vi "Elevator Settled.vi"(8 "error in (no error)":errorcluster, 10 "State":T1=enum."Tote 1", 11 "Elevator Inputs":T2={"Up"=FALSE, "Down"=FALSE, "Bin Modifier"=FALSE, "Pickup"=FALSE, "Top LS"=FALSE, "Bottom LS"=FALSE, "Encoder Position"=-460.0, "Encoder Velocity"=0.0, "Manual Control"=0.0}) -> (0 "error out":errorcluster, 2 "Settled?":bool, 3 "State":T1=enum."Tote 1")   [LabVIEW 2014]
uses:
  Elevator Input Data.ctl
  Elevator States.ctl
panel:
  in  "Velocity\nTolerance":dbl=300000000.0
  in  "Position\nTolerance":dbl=50.0
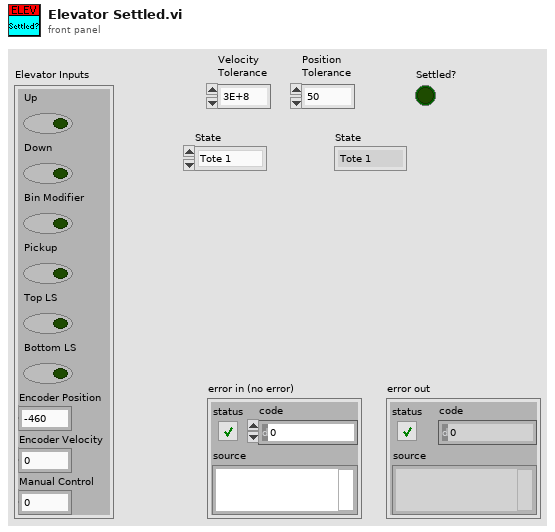
[diagram p1: front panel]
types:
  T1 = typedef "Elevator States.ctl" = enum16{"Ground", "Tote 1", "Tote 2", "Tote 3", "Tote 4", "Tote 5", "Tote 6"}
  T2 = typedef "Elevator Input Data.ctl" = cluster{"Up":bool, "Down":bool, "Bin Modifier":bool, "Pickup":bool, "Top LS":bool, "Bottom LS":bool, "Encoder Position":dbl, "Encoder Velocity":dbl, "Manual Control":dbl}
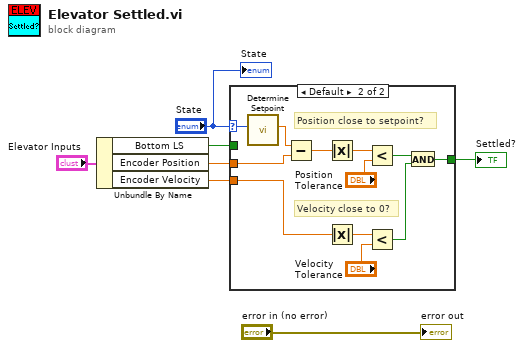
[diagram p0: block diagram]
diagram:
  n1 = Unbundle By Name("Elevator Inputs") -> ("Bottom LS"=w6:bool, "Encoder Position"=w5:dbl, "Encoder Velocity"=w4:dbl)
  n2 = case shown="Default" "State" {
    selector: "State" -> [_ w10]
    tunnel: [w8 w11] -> w2
    tunnel: w5 -> [_ w19]
    tunnel: w4 -> [_ w18]
    tunnel: w6 -> [w8 _]
    frame "Ground" {
    }
    frame Default {
      # "Position close to setpoint?"
      # "Velocity close to 0?"
      n3 = call "Determine Setpoint.vi"("Elevator State"=w10) -> ("Setpoint"=w9:dbl)  [unwired: 9 in, 1 out]
      n4 = Subtract(x=w9, y=w19) -> (x-y=w20:dbl)
      n5 = Absolute Value(x=w20) -> (abs(x)=w17:dbl)
      n6 = Absolute Value(x=w18) -> (abs(x)=w16:dbl)
      n7 = Less?(x=w17, y="Position\nTolerance") -> (x < y?=w13:bool)
      n8 = Less?(x=w16, y="Velocity\nTolerance") -> (x < y?=w12:bool)
      n9 = And(x=w13, y=w12) -> (x .and. y?=w11:bool)
    }
  }
  "Settled?" <- w2
  "error out" <- "error in (no error)"
  "State" <- "State"
